vi "Cond Broadcast.vi"(8 "error in (no error)":errorcluster, 11 "Cond in":T1) -> (0 "error out":errorcluster, 3 "Cond out":T1)   [LabVIEW 2013, in "Linux RT IPC.lvlib" / "POSIX Threads.lvlib" / "Cond.lvclass"]
doc: "Calls pthread_cond_broadcast() on the pthread cond object encapsulated by Cond.\n\nRefer to online POSIX documentation for more information."
uses:
  Cond.lvclass
  Controls/reference.ctl
  POSIX Thread Object/POSIX Thread Object.lvclass/POSIX Thread Object.ctl
  POSIX Thread Object/Private VIs/libpthread path.vi
  POSIX Thread Object/Private VIs/get pthread error.vi
  POSIX Thread Object/POSIX Thread Object.lvclass
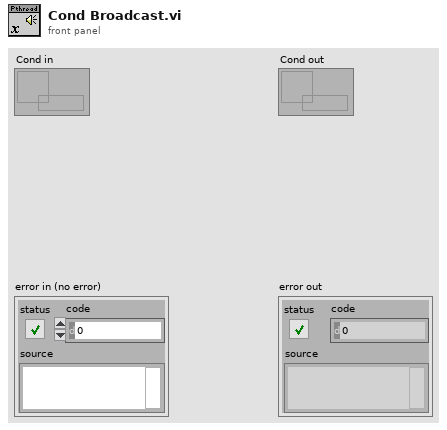
[diagram p1: front panel]
types:
  T1 = typedef "Linux RT IPC.lvlib/POSIX Threads.lvlib/Cond.lvclass/reference.ctl" = refnum<data-value>
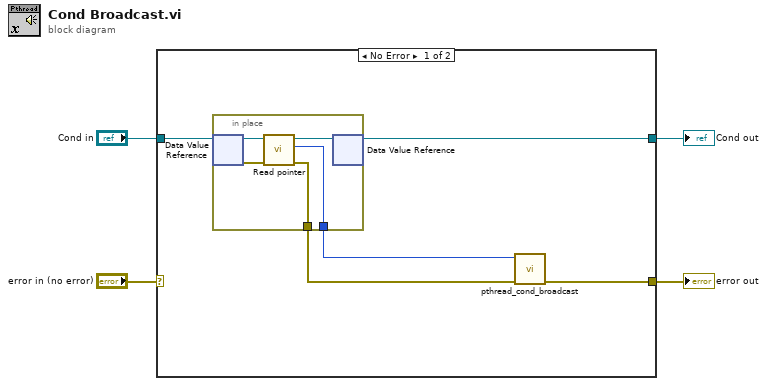
[diagram p0: block diagram]
diagram:
  n1 = case shown="No Error" "error in (no error)" {
    selector: "error in (no error)" -> [_ w16]
    tunnel: [w9 w16] -> w3
    tunnel: "Cond in" -> [w8 w15]
    tunnel: [w7 w15] -> w2
    frame No Error {
      n2 = in-place {
        in-place-border: [w11] -> w6
        in-place-border: [w10] -> w5
        n3 = in-place-dvr #1(w8) -> (w14:refnum<class "Cond.lvclass">, w12:errorcluster)
        n4 = call "Read pointer.vi"("error in (no error)"=w12, "POSIX Thread Object in"=w14) -> ("error out"=w11:errorcluster, "pointer"=w10:u64, "POSIX Thread Object out"=w13:refnum<class "Cond.lvclass">)  [unwired: 7 in]
        n5 = in-place-dvr #1(w13) -> (w7:T1)  [unwired: 1 out]
      }
      n6 = call "pthread_cond_broadcast.vi"("error in (no error)"=w6, "cond ptr in"=w5) -> ("error out"=w9:errorcluster)  [unwired: 8 in, 1 out]
    }
    frame Error {
    }
  }
  "Cond out" <- w2
  "error out" <- w3
